vi "Main On Compile Action VI - Multi FPGA.vi"(8 "error in (no error)":errorcluster, 11 "Device Item Ref in":T26 format="%.0x") -> (0 "error out":errorcluster)   [LabVIEW 2015, in "Engine Simulation Toolkit System Explorer.lvlib"]
uses:
  Engine Simulation Toolkit System Explorer.lvlib
  <vilib>/NI Veristand/Custom Device API/Custom Device Item Ref.ctl
  FPGA Datum.ctl
  Shared/1.0 APU Engine Data.ctl
  Shared/1.0 APU Engine FIFO Idxs.ctl
  Shared/1.0 Digital Pattern Gen Engine Data.ctl
  Shared/1.0 Digital Pattern Gen FIFO Idxs.ctl
  Shared/1.0 Event Timing Capture Engine Data.ctl
  Shared/1.0 Event Timing Capture FIFO Idxs.ctl
  Shared/1.1 APU Engine Data.ctl
  Shared/1.0 Directional Speed Engine Data.ctl
  Shared/1.0 Directional Speed FIFO Idxs.ctl
  Shared/1.0 Analog Replay Engine Data.ctl
  Shared/1.0 Analog Replay FIFO Idxs.ctl
  Shared/1.0 Event Timing Measure Engine Data.ctl
  Shared/1.0 Event Timing Measure FIFO Idxs.ctl
  Shared/1.0 Knock Sensor Engine Data.ctl
  Shared/1.0 Knock Sensor FIFO Idxs.ctl
  Shared/1.0 Knock Cylinder Engine Data.ctl
  Shared/1.0 Knock Cylinder FIFO Idxs.ctl
  Shared/1.1 Event Timing Measure Engine Data.ctl
  Shared/1.3 Digital Pattern Gen Engine Data.ctl
  Shared/1.3 Digital Pattern Gen FIFO Idxs.ctl
  Shared/Bitfile EST Version.ctl
  Shared/1.3 APU Engine Data.ctl
  Shared/Engine Init Data.ctl
  Shared/Engine Status Data.ctl
  Shared/Compiled Data.ctl
  Shared/Properties.vi
  <vilib>/NI Veristand/Custom Device API/Set Item Property (Variant).vi
  <vilib>/NI Veristand/Custom Device API/Get Item Property (String Array).vi
  <vilib>/NI Veristand/Custom Device API/Custom Device API.lvlib
  Shared/Engine Simulation Toolkit Shared.lvlib
panel:
  out "Status":T1
  out "System":T2
  out "Array":T3[](array[typedef]) {"1.1 APUs"."shared settings"."cycle start" format="%#.15g"; "1.0 APUs"."shared settings"."cycle start" format="%#.15g"}
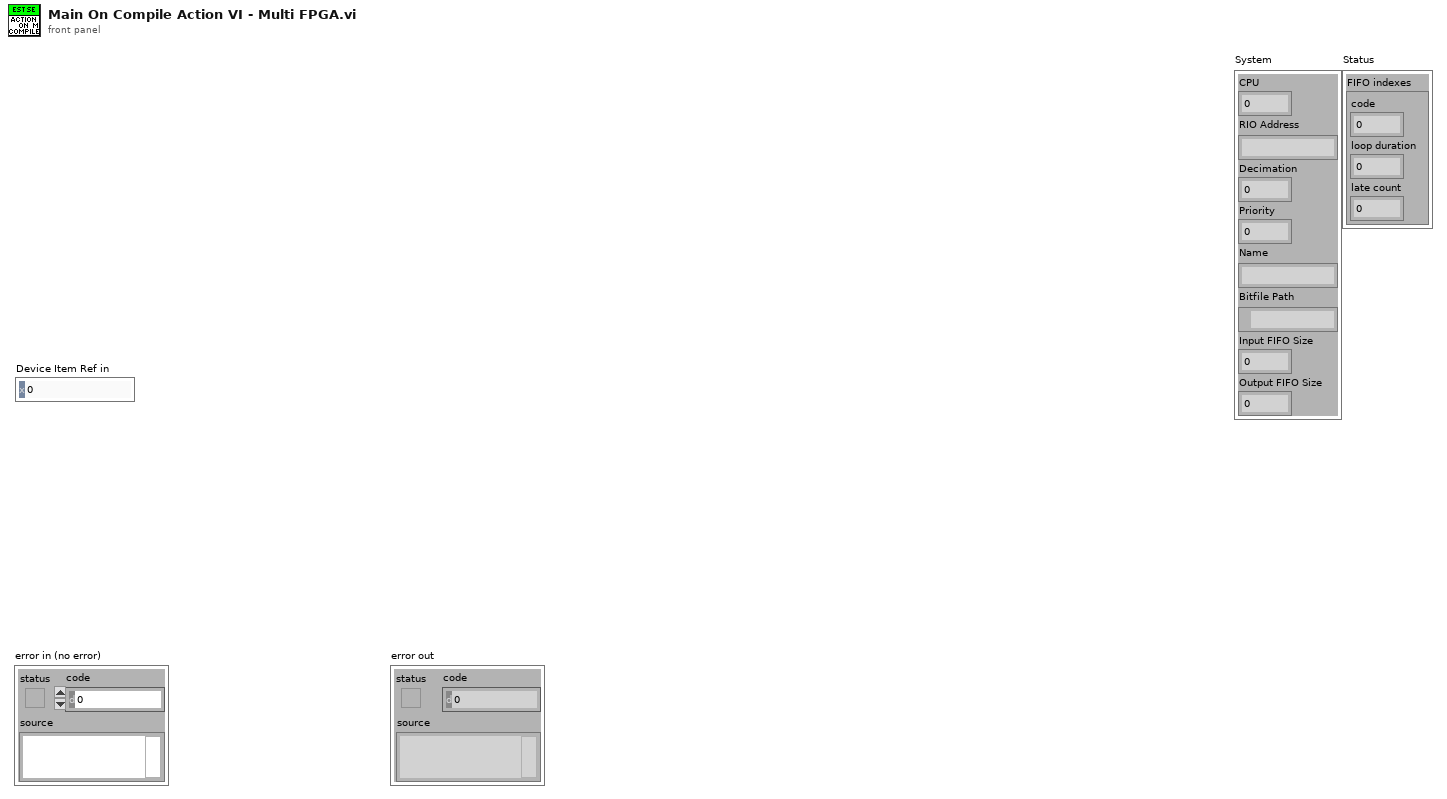
[diagram p1: front panel]
types:
  T1 = typedef "Engine Simulation Toolkit Shared.lvlib/Engine Status Data.ctl" = cluster{"FIFO indexes":cluster{"code":i32, "loop duration":i32, "late count":i32}}
  T2 = typedef "Engine Simulation Toolkit Shared.lvlib/Engine Init Data.ctl" = cluster{"CPU":i32, "RIO Address":string, "Decimation":i64, "Priority":i32, "Name":string, "Bitfile Path":path, "Input FIFO Size":i32, "Output FIFO Size":i32}
  T3 = typedef "Engine Simulation Toolkit Shared.lvlib/FPGA Datum.ctl" = cluster{"Bitfile Path":path, "RIO Address":string, "1.0 APUs":T4[], "Unused Analog Replays":string[], "1.0 Digital Pattern Gens":T6[], "Unused Digital Pattern Gens":string[], "1.0 Event Captures":T8[], "Unused Directional Sensors":string[], "1.1 APUs":T10[], "1.0 Directional Speed":T11[], "1.0 Analog Replays":T13[], "1.0 Event Measures":T15[], "1.0 Knock Sensors":T17[], "1.0 Knock Cylinders":T19[], "1.1 Event Measures":T21[], "1.3 Digital Pattern Gens":T22[], "Bitfile EST Version":T24, "1.3 APUs":T25[]}
  T4 = typedef "Engine Simulation Toolkit Shared.lvlib/1.0 APU Engine Data.ctl" = cluster{"register names":cluster{"shared settings":string, "input":string, "settings":string, "output":string}, "shared settings":cluster{"cycle start":fxp<+,2,2>, "crank start":u16, "stuck limit":fxp<+,18,18>}, "settings":cluster{"acceleration":fxp<+,18,-20>, "max cycle":fxp<+,2,2>, "enable accel":bool}, "FIFO indexes":T5, "input":cluster{"desired speed":fxp<+/-,23,2>, "reset":bool}, "degrees of 1 cycle u16":dbl, "degrees of 1 crank u16":dbl}
  T5 = typedef "Engine Simulation Toolkit Shared.lvlib/1.0 APU Engine FIFO Idxs.ctl" = cluster{"inputs":cluster{"desired speed":i32, "reset":i32}, "outputs":cluster{"crank angle":i32, "cycle angle":i32, "actual speed":i32}}
  T6 = typedef "Engine Simulation Toolkit Shared.lvlib/1.0 Digital Pattern Gen Engine Data.ctl" = cluster{"register names":cluster{"load input":string, "settings":string, "input":string}, "settings":cluster{"edge 1":u16, "edge 2":u16, "cycle angle":bool, "enabled":bool, "first falling":bool}, "FIFO indexes":T7, "input":cluster{"Offset":i16}, "offset convert":dbl, "Position LUT":u16[]}
  T7 = typedef "Engine Simulation Toolkit Shared.lvlib/1.0 Digital Pattern Gen FIFO Idxs.ctl" = cluster{"offset":i32}
  T8 = typedef "Engine Simulation Toolkit Shared.lvlib/1.0 Event Timing Capture Engine Data.ctl" = cluster{"register names":cluster{"output":string}, "FIFO indexes":T9, "degrees of 1 u16":dbl, "wrap":bool, "window min":u16, "duration convert":dbl, "default start":dbl, "default end":dbl, "ref angle":dbl}
  T9 = typedef "Engine Simulation Toolkit Shared.lvlib/1.0 Event Timing Capture FIFO Idxs.ctl" = cluster{"start angle":i32, "end angle":i32, "duration":i32}
  T10 = typedef "Engine Simulation Toolkit Shared.lvlib/1.1 APU Engine Data.ctl" = cluster{"register names":cluster{"shared settings":string, "input":string, "settings":string, "output":string, "go":string}, "shared settings":cluster{"cycle start":fxp<+,2,2>, "crank start":u16, "stuck limit":fxp<+,18,18>}, "settings":cluster{"acceleration":fxp<+,18,-20>, "max cycle":fxp<+,2,2>, "enable accel":bool}, "FIFO indexes":T5, "input":cluster{"desired speed":fxp<+/-,23,2>, "reset":bool}, "degrees of 1 cycle u16":dbl, "degrees of 1 crank u16":dbl}
  T11 = typedef "Engine Simulation Toolkit Shared.lvlib/1.0 Directional Speed Engine Data.ctl" = cluster{"register names":cluster{"settings":string, "input":string, "load input":string}, "settings":cluster{"Upper Value":u16, "Lower Value":u16, "Upper Index":fxp<+,10,10>, "Lower Index":fxp<+,10,10>, "Enabled":bool}, "input":cluster{"td (tics)":u16, "tf (tics)":u16, "tr (tics)":u16}, "FIFO indexes":T12, "Tooth Centers LUT":u16[]}
  T12 = typedef "Engine Simulation Toolkit Shared.lvlib/1.0 Directional Speed FIFO Idxs.ctl" = cluster{"td":i32, "tf":i32, "tr":i32}
  T13 = typedef "Engine Simulation Toolkit Shared.lvlib/1.0 Analog Replay Engine Data.ctl" = cluster{"register names":cluster{"load input":string, "settings":string, "input":string}, "settings":cluster{"ReverseNegate":bool, "CycleAngle":bool, "SpeedThreshold":fxp<+/-,23,2>, "AOBelowThreshold":i16}, "FIFO indexes":T14, "input":cluster{"Offset":i16, "VScaleSlope":fxp<+,18,6>, "VScaleIntercept":fxp<+/-,18,3>}, "offset convert":dbl, "DAC LUT":i16[], "SE_VScaleIntercept":fxp<+/-,18,3>, "SE_VScaleSlope":fxp<+,18,6>, "VOverride":bool, "ResetVolts":bool}
  T14 = typedef "Engine Simulation Toolkit Shared.lvlib/1.0 Analog Replay FIFO Idxs.ctl" = cluster{"enable voltage":i32, "volt slope":i32, "volt intercept":i32, "offset":i32}
  T15 = typedef "Engine Simulation Toolkit Shared.lvlib/1.0 Event Timing Measure Engine Data.ctl" = cluster{"register names":cluster{"settings":string, "output":string}, "settings":cluster{"max":u16, "min":u16, "active high":bool, "wrap":bool, "full window":bool}, "FIFO indexes":T16}
  T16 = typedef "Engine Simulation Toolkit Shared.lvlib/1.0 Event Timing Measure FIFO Idxs.ctl" = cluster{"stuck active":i32, "win all active":i32, "win orph start":i32, "win orph end":i32}
  T17 = typedef "Engine Simulation Toolkit Shared.lvlib/1.0 Knock Sensor Engine Data.ctl" = cluster{"register names":cluster{"settings":string, "input":string}, "settings":cluster{"low freq (periods/tick)":fxp<+,32,0>, "high freq (periods/tick)":fxp<+,32,0>, "duration (1.25MHz tics)":fxp<+,18,18>, "low freq speed slope":fxp<+,16,-3>, "low freq speed intercept":fxp<+,10,-10>, "low freq by speed":bool}, "DAC multiplier":dbl, "FIFO indexes":T18, "input":cluster{"low freq scaler":fxp<+,10,0>}}
  T18 = typedef "Engine Simulation Toolkit Shared.lvlib/1.0 Knock Sensor FIFO Idxs.ctl" = cluster{"amp":i32}
  T19 = typedef "Engine Simulation Toolkit Shared.lvlib/1.0 Knock Cylinder Engine Data.ctl" = cluster{"register names":cluster{"settings":string, "input":string}, "settings":cluster{"seed":u16, "reset":bool}, "input":cluster{"probability compare":u16, "high freq scaler":fxp<+,10,0>, "trigger position":u16}, "DAC multiplier":dbl, "FIFO indexes":T20, "Angle multiplier":dbl}
  T20 = typedef "Engine Simulation Toolkit Shared.lvlib/1.0 Knock Cylinder FIFO Idxs.ctl" = cluster{"prob":i32, "amp":i32, "pos":i32}
  T21 = typedef "Engine Simulation Toolkit Shared.lvlib/1.1 Event Timing Measure Engine Data.ctl" = cluster{"register names":cluster{"settings":string, "output":string}, "settings":cluster{"max":u16, "min":u16, "active high":bool, "wrap":bool}, "FIFO indexes":T16}
  T22 = typedef "Engine Simulation Toolkit Shared.lvlib/1.3 Digital Pattern Gen Engine Data.ctl" = cluster{"register names":cluster{"load input":string, "settings":string, "input":string}, "settings":cluster{"edge 1":u16, "edge 2":u16, "cycle angle":bool, "enabled":bool, "first falling":bool, "fault":bool, "fault wrap":bool, "fault value":bool, "fault count":fxp<+,4,4>, "use fault count":bool}, "FIFO indexes":T23, "input":cluster{"Offset":i16}, "deg to u16 scale":dbl, "Position LUT":u16[], "# of teeth":i16, "max angle":dbl}
  T23 = typedef "Engine Simulation Toolkit Shared.lvlib/1.3 Digital Pattern Gen FIFO Idxs.ctl" = cluster{"offset":i32, "command":i32, "rotations":i32, "start angle":i32, "stop angle":i32, "tooth to rem":i32, "trigger":i32, "valid":i32}
  T24 = typedef "Engine Simulation Toolkit Shared.lvlib/Bitfile EST Version.ctl" = enum16{"1.0", "1.1", "1.2", "1.3", "1.4"}
  T25 = typedef "Engine Simulation Toolkit Shared.lvlib/1.3 APU Engine Data.ctl" = cluster{"register names":cluster{"shared settings":string, "input":string, "settings":string, "output":string, "go":string}, "shared settings":cluster{"start":fxp<+,17,17>, "stuck limit":fxp<+,18,18>}, "settings":cluster{"acceleration":fxp<+,18,-20>, "enable accel":bool}, "FIFO indexes":T5, "input":cluster{"desired speed":fxp<+/-,23,2>, "reset":bool}, "degrees of 1 cycle u16":dbl, "degrees of 1 crank u16":dbl}
  T26 = typedef "Custom Device API.lvlib/Custom Device Item Ref.ctl" = u64
  T27 = typedef "Engine Simulation Toolkit Shared.lvlib/Compiled Data.ctl" = cluster{"Init":T2, "1.0 APUs":T4[], "Status":T1, "DevOutFIFO":refnum<k33>, "DevInFIFO":refnum<k33>, "Device Inputs":dbl[], "Device Outputs":dbl[], "Last Device Inputs":dbl[], "1.0 Analog Replays":T13[], "Unused Analog Replays":string[], "1.0 Digital Pattern Gens":T6[], "Unused Digital Pattern Gens":string[], "1.0 Event Captures":T8[], "1.0 Event Measures":T15[], "1.0 Knock Sensors":T17[], "1.0 Knock Cylinders":T19[], "1.0 Directional Speed":T11[], "Unused Directional Sensors":string[], "1.1 APUs":T10[], "1.1 Event Measures":T21[], "1.3 Digital Pattern Gens":T22[], "Bitfile EST Version":T24, "1.3 APUs":T25[], "Feature Toggles":cluster{"Multi FPGA":bool}, "FPGA Data":T3[]}
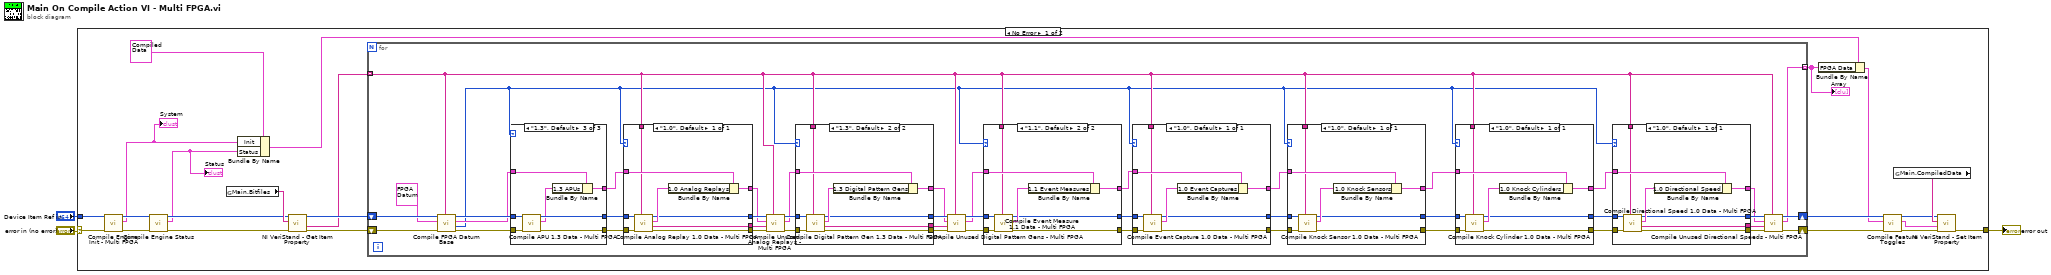
[diagram p0: block diagram]
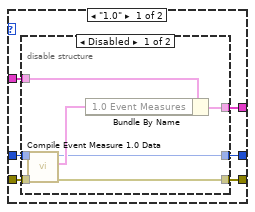
[diagram p2: hidden frame]
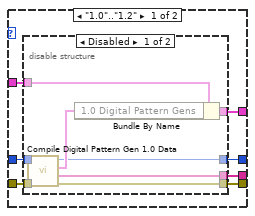
[diagram p4: hidden frame]
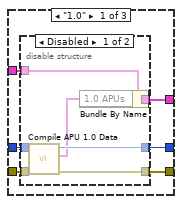
[diagram p6: hidden frame]
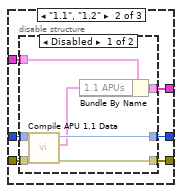
[diagram p8: hidden frame]
diagram:
  n1 = case shown="No Error" "error in (no error)" {
    selector: "error in (no error)" -> [w15 w203]
    tunnel: [w26 w203] -> w2
    tunnel: "Device Item Ref in" -> [w16 _]
    frame No Error {
      n2 = call "Compile Engine Init - Multi FPGA.vi"("error in (no error)"=w15, "Device Item Ref in"=w16) -> ("error out"=w11:errorcluster, "System"=w7:T2, "Device Item Ref out"=w12:T26)  [unwired: 7 in]
      "System" <- w7
      n3 = call "Compile Engine Status.vi"("error in (no error)"=w11, "Device Item Ref in"=w12) -> ("error out"=w10:errorcluster, "Status"=w8:T1, "Device Item Ref out"=w9:T26)  [unwired: 7 in]
      "Status" <- w8
      n4 = global read "Properties.vi" "Main.Bitfiles"() -> (w20:string)
      n5 = Bundle By Name(cluster=T27 {"Init"={"CPU"=0, "RIO Address"="", "Decimation"=0, "Priority"=0, "Name"="", "Bitfile Path"=path "", "Input FIFO Size"=0, "Output FIFO Size"=0}, "1.0 APUs"=[], "Status"={"FIFO indexes"={"code"=0, "loop duration"=0, "late count"=0}}, "DevOutFIFO"=refnum, "DevInFIFO"=refnum, "Device Inputs"=[], "Device Outputs"=[], "Last Device Inputs"=[], "1.0 Analog Replays"=[], "Unused Analog Replays"=[], "1.0 Digital Pattern Gens"=[], "Unused Digital Pattern Gens"=[], "1.0 Event Captures"=[], "1.0 Event Measures"=[], "1.0 Knock Sensors"=[], "1.0 Knock Cylinders"=[], "1.0 Directional Speed"=[], "Unused Directional Sensors"=[], "1.1 APUs"=[], "1.1 Event Measures"=[], "1.3 Digital Pattern Gens"=[], "Bitfile EST Version"=enum."1.0", "1.3 APUs"=[], "Feature Toggles"={"Multi FPGA"=FALSE}, "FPGA Data"=[]} ("Compiled Data"), "Init"=w7, "Status"=w8) -> (w6:T27)
      n6 = call-poly <vilib>:"NI VeriStand - Get Item Property.vi"("error in (no error)"=w10, "Property Name"=w20, "Item Ref in"=w9) -> ("error out"=w19:errorcluster, "Value"=w17:string[], "Item Ref out"=w18:T26)  [unwired: 5 in, 1 out]
      n7 = for {
        tunnel: w17 -> [w29] mode=indexing
        shift-right: [w70] -> w24
        shift-left: w19 -> [w68]
        shift-right: [w69] -> w23
        shift-left: w18 -> [w31]
        tunnel: [w34] -> w5 mode=indexing
        n8 = call "Compile FPGA Datum Base.vi"("RIO Address"=w29, "error in (no error)"=w68, "FPGA Datum in"=T3 {"Bitfile Path"=path "", "RIO Address"="", "1.0 APUs"=[], "Unused Analog Replays"=[], "1.0 Digital Pattern Gens"=[], "Unused Digital Pattern Gens"=[], "1.0 Event Captures"=[], "Unused Directional Sensors"=[], "1.1 APUs"=[], "1.0 Directional Speed"=[], "1.0 Analog Replays"=[], "1.0 Event Measures"=[], "1.0 Knock Sensors"=[], "1.0 Knock Cylinders"=[], "1.1 Event Measures"=[], "1.3 Digital Pattern Gens"=[], "Bitfile EST Version"=enum."1.0", "1.3 APUs"=[]} ("FPGA Datum"), "Item Ref in"=w31) -> ("error out"=w37:errorcluster, "EST version enum"=w27:T24, "FPGA Datum out"=w28:T3, "Item Ref out"=w32:T26)  [unwired: 4 in]
        n9 = case shown="\"1.3\", Default" w27 {
          tunnel: w37 -> [w169 w185 w202]
          tunnel: [w168 w184 w201] -> w66
          tunnel: w32 -> [w167 w183 w200]
          tunnel: [w166 w182 w199] -> w65
          tunnel: w28 -> [w165 w181 w198]
          tunnel: [w164 w180 w197] -> w67
          frame "1.0" {
            n10 = disable-structure shown="Disabled" {
              disable-tunnel: w169 -> [w176 w179]
              disable-tunnel: [w175 w179] -> w168
              disable-tunnel: w167 -> [w174 w178]
              disable-tunnel: [w173 w178] -> w166
              disable-tunnel: w165 -> [w172 w177]
              disable-tunnel: [w170 w177] -> w164
              frame Disabled {
                n11 = call "Compile APU 1.0 Data.vi"("error in (no error)"=w176, "Device Item Ref in"=w174) -> ("error out"=w175:errorcluster, "APUs"=w171:T4[], "Device Item Ref out"=w173:T26)  [unwired: 7 in]
                n12 = Bundle By Name(cluster=w172, "1.0 APUs"=w171) -> (w170:T3)
              }
              frame Enabled {
              }
            }
          }
          frame "1.1", "1.2" {
            n13 = disable-structure shown="Disabled" {
              disable-tunnel: w185 -> [w192 w193]
              disable-tunnel: [w191 w193] -> w184
              disable-tunnel: w183 -> [w190 w194]
              disable-tunnel: [w189 w194] -> w182
              disable-tunnel: w181 -> [w188 w195]
              disable-tunnel: [w187 w195] -> w180
              frame Disabled {
                n14 = call "Compile APU 1.1 Data.vi"("error in (no error)"=w192, "Device Item Ref in"=w190) -> ("error out"=w191:errorcluster, "APUs"=w186:T10[], "Device Item Ref out"=w189:T26)  [unwired: 7 in]
                n15 = Bundle By Name(cluster=w188, "1.1 APUs"=w186) -> (w187:T3)
              }
              frame Enabled {
              }
            }
          }
          frame "1.3", Default {
            n16 = call "Compile APU 1.3 Data - Multi FPGA.vi"("error in (no error)"=w202, "Device Item Ref in"=w200) -> ("error out"=w201:errorcluster, "APUs"=w196:T25[], "Device Item Ref out"=w199:T26)  [unwired: 7 in]
            n17 = Bundle By Name(cluster=w198, "1.3 APUs"=w196) -> (w197:T3)
          }
        }
        n18 = case shown="\"1.0\", Default" w27 {
          tunnel: [w158] -> w64
          tunnel: w65 -> [w163]
          tunnel: [w157] -> w63
          tunnel: w67 -> [w162]
          tunnel: [w160] -> w35
          tunnel: w66 -> [w159]
          tunnel: [w156] -> w62
          tunnel: w29 -> [w155]
          frame "1.0", Default {
            n19 = call "Compile Analog Replay 1.0 Data - Multi FPGA.vi"("RIO Address"=w155, "error in (no error)"=w159, "Device Item Ref in"=w163) -> ("error out"=w158:errorcluster, "bitfile names"=w156:string[], "Analog Replays"=w161:T13[], "Device Item Ref out"=w157:T26)  [unwired: 5 in]
            n20 = Bundle By Name(cluster=w162, "1.0 Analog Replays"=w161) -> (w160:T3)
          }
        }
        n21 = call "Compile Unused Analog Replays - Multi FPGA.vi"("RIO Address"=w29, "error in (no error)"=w64, "bitfile names"=w62, "FPGA Datum in"=w35, "Device Item Ref in"=w63) -> ("error out"=w60:errorcluster, "FPGA Datum out"=w59:T3, "Item Ref out"=w61:T26)  [unwired: 4 in]
        n22 = case shown="\"1.3\", Default" w27 {
          tunnel: [w130 w149] -> w58
          tunnel: w61 -> [w134 w154]
          tunnel: [w129 w148] -> w56
          tunnel: w59 -> [w133 w153]
          tunnel: [w132 w151] -> w36
          tunnel: w60 -> [w131 w150]
          tunnel: [w128 w147] -> w57
          tunnel: w29 -> [_ w146]
          frame "1.0".."1.2" {
            n23 = disable-structure shown="Disabled" {
              disable-tunnel: w134 -> [w142 w144]
              disable-tunnel: w133 -> [w141 w145]
              disable-tunnel: [w139 w145] -> w132
              disable-tunnel: w131 -> [w138 w143]
              disable-tunnel: [w137 w143] -> w130
              disable-tunnel: [w136 w144] -> w129
              disable-tunnel: [w135 _] -> w128
              frame Disabled {
                n24 = call "Compile Digital Pattern Gen 1.0 Data.vi"("error in (no error)"=w138, "Device Item Ref in"=w142) -> ("error out"=w137:errorcluster, "bitfile names"=w135:string[], "Digital Pattern Gens"=w140:T6[], "Device Item Ref out"=w136:T26)  [unwired: 6 in]
                n25 = Bundle By Name(cluster=w141, "1.0 Digital Pattern Gens"=w140) -> (w139:T3)
              }
              frame Enabled {
              }
            }
          }
          frame "1.3", Default {
            n26 = call "Compile Digital Pattern Gen 1.3 Data - Multi FPGA.vi"("RIO Address"=w146, "error in (no error)"=w150, "Device Item Ref in"=w154) -> ("error out"=w149:errorcluster, "bitfile names"=w147:string[], "Digital Pattern Gens"=w152:T22[], "Device Item Ref out"=w148:T26)  [unwired: 5 in]
            n27 = Bundle By Name(cluster=w153, "1.3 Digital Pattern Gens"=w152) -> (w151:T3)
          }
        }
        n28 = call "Compile Unused Digital Pattern Gens - Multi FPGA.vi"("RIO Address"=w29, "error in (no error)"=w58, "bitfile names"=w57, "FPGA Datum in"=w36, "Device Item Ref in"=w56) -> ("error out"=w55:errorcluster, "FPGA Datum out"=w53:T3, "Item Ref out"=w54:T26)  [unwired: 4 in]
        n29 = case shown="\"1.1\", Default" w27 {
          tunnel: [w105 w122] -> w50
          tunnel: w54 -> [w109 w127]
          tunnel: [w104 w121] -> w52
          tunnel: w53 -> [w108 w126]
          tunnel: [w107 w124] -> w51
          tunnel: w55 -> [w106 w123]
          tunnel: w29 -> [_ w120]
          frame "1.0" {
            n30 = disable-structure shown="Disabled" {
              disable-tunnel: w109 -> [w116 w118]
              disable-tunnel: w108 -> [w115 w119]
              disable-tunnel: [w113 w119] -> w107
              disable-tunnel: w106 -> [w112 w117]
              disable-tunnel: [w111 w117] -> w105
              disable-tunnel: [w110 w118] -> w104
              frame Disabled {
                n31 = call "Compile Event Measure 1.0 Data.vi"("error in (no error)"=w112, "Device Item Ref in"=w116) -> ("error out"=w111:errorcluster, "Event Timing Measures"=w114:T15[], "Device Item Ref out"=w110:T26)  [unwired: 7 in]
                n32 = Bundle By Name(cluster=w115, "1.0 Event Measures"=w114) -> (w113:T3)
              }
              frame Enabled {
              }
            }
          }
          frame "1.1", Default {
            n33 = call "Compile Event Measure 1.1 Data - Multi FPGA.vi"("RIO Address"=w120, "error in (no error)"=w123, "Device Item Ref in"=w127) -> ("error out"=w122:errorcluster, "Event Timing Measures"=w125:T21[], "Device Item Ref out"=w121:T26)  [unwired: 6 in]
            n34 = Bundle By Name(cluster=w126, "1.1 Event Measures"=w125) -> (w124:T3)
          }
        }
        n35 = case shown="\"1.0\", Default" w27 {
          tunnel: [w98] -> w47
          tunnel: w52 -> [w103]
          tunnel: [w97] -> w48
          tunnel: w51 -> [w102]
          tunnel: [w100] -> w49
          tunnel: w50 -> [w99]
          tunnel: w29 -> [w96]
          frame "1.0", Default {
            n36 = call "Compile Event Capture 1.0 Data - Multi FPGA.vi"("RIO Address"=w96, "error in (no error)"=w99, "Device Item Ref in"=w103) -> ("error out"=w98:errorcluster, "Event Timing Captures"=w101:T8[], "Device Item Ref out"=w97:T26)  [unwired: 6 in]
            n37 = Bundle By Name(cluster=w102, "1.0 Event Captures"=w101) -> (w100:T3)
          }
        }
        n38 = case shown="\"1.0\", Default" w27 {
          tunnel: [w90] -> w45
          tunnel: w48 -> [w95]
          tunnel: [w89] -> w46
          tunnel: w49 -> [w94]
          tunnel: [w92] -> w44
          tunnel: w47 -> [w91]
          tunnel: w29 -> [w88]
          frame "1.0", Default {
            n39 = call "Compile Knock Sensor 1.0 Data - Multi FPGA.vi"("RIO Address"=w88, "error in (no error)"=w91, "Device Item Ref in"=w95) -> ("error out"=w90:errorcluster, "Knock Sensors"=w93:T17[], "Device Item Ref out"=w89:T26)  [unwired: 6 in]
            n40 = Bundle By Name(cluster=w94, "1.0 Knock Sensors"=w93) -> (w92:T3)
          }
        }
        n41 = case shown="\"1.0\", Default" w27 {
          tunnel: [w82] -> w39
          tunnel: w46 -> [w87]
          tunnel: [w81] -> w38
          tunnel: w44 -> [w86]
          tunnel: [w84] -> w40
          tunnel: w45 -> [w83]
          tunnel: w29 -> [w80]
          frame "1.0", Default {
            n42 = call "Compile Knock Cylinder 1.0 Data - Multi FPGA.vi"("RIO Address"=w80, "error in (no error)"=w83, "Device Item Ref in"=w87) -> ("error out"=w82:errorcluster, "Knock Cylinders"=w85:T19[], "Device Item Ref out"=w81:T26)  [unwired: 6 in]
            n43 = Bundle By Name(cluster=w86, "1.0 Knock Cylinders"=w85) -> (w84:T3)
          }
        }
        n44 = case shown="\"1.0\", Default" w27 {
          tunnel: [w74] -> w41
          tunnel: w38 -> [w79]
          tunnel: [w73] -> w43
          tunnel: w40 -> [w78]
          tunnel: [w76] -> w33
          tunnel: w39 -> [w75]
          tunnel: [w72] -> w42
          tunnel: w29 -> [w71]
          frame "1.0", Default {
            n45 = call "Compile Directional Speed 1.0 Data - Multi FPGA.vi"("RIO Address"=w71, "error in (no error)"=w75, "Device Item Ref in"=w79) -> ("error out"=w74:errorcluster, "bitfile names"=w72:string[], "Directional Speeds"=w77:T11[], "Device Item Ref out"=w73:T26)  [unwired: 5 in]
            n46 = Bundle By Name(cluster=w78, "1.0 Directional Speed"=w77) -> (w76:T3)
          }
        }
        n47 = call "Compile Unused Directional Speeds - Multi FPGA.vi"("RIO Address"=w29, "error in (no error)"=w41, "bitfile names"=w42, "FPGA Datum in"=w33, "Device Item Ref in"=w43) -> ("error out"=w70:errorcluster, "FPGA Datum out"=w34:T3, "Item Ref out"=w69:T26)  [unwired: 4 in]
      }
      "Array" <- w5
      n48 = Bundle By Name(cluster=w6, "FPGA Data"=w5) -> (w14:T27)
      n49 = call "Compile Feature Toggles.vi"("error in (no error)"=w24, "Compiled Data in"=w14, "Device Item Ref in"=w23) -> ("error out"=w4:errorcluster, "Compiled Data out"=w22:T27, "Item Ref out"=w21:T26)  [unwired: 6 in]
      n50 = global read "Properties.vi" "Main.CompiledData"() -> (w25:string)
      n51 = call-poly <vilib>:"NI VeriStand - Set Item Property.vi"("error in (no error)"=w4, "Value"=w22, "Property Name"=w25, "Item Ref in"=w21) -> ("error out"=w26:errorcluster)  [unwired: 5 in, 2 out]
    }
    frame Error {
    }
  }
  "error out" <- w2
